vi "Map.vi"(7 "Action":enum8{"noop", "get", "set", "pop"}(ring), 9 "Is Registered in":bool, 10 "User Event in":refnum<user-event>, 11 "User Event Name":string) -> (0 "Found?":bool, 1 "Is Registered out":bool, 2 "User Event out":refnum<user-event>)   [LabVIEW 2018, in "UserEvent.lvlib"]
uses:
  UserEvent.lvlib
panel:
  # "Missing object. The object \"Map\" does not exist in the previous version."
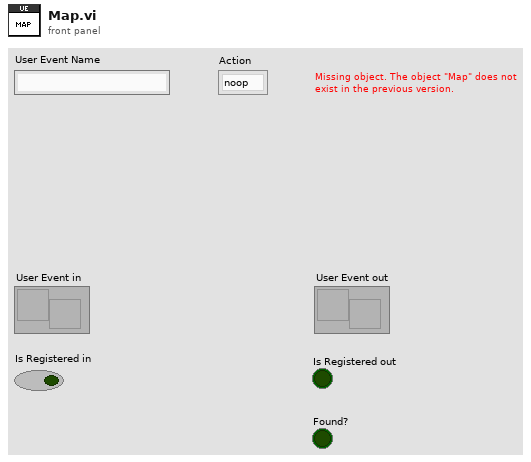
[diagram p1: front panel]
types:
  T1 = cluster{"User Event in":refnum<user-event>, "Is Registered in":bool}
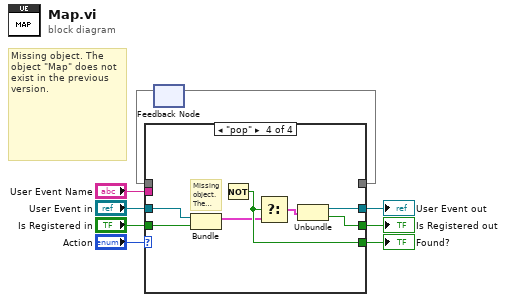
[diagram p0: block diagram]
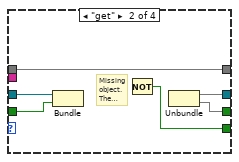
[diagram p3: hidden frame]
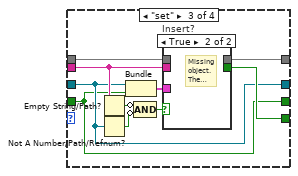
[diagram p4: hidden frame]
diagram:
  # "Missing object. The object \"Map\" does not exist in the previous version."
  n1 = feedback #1() -> (w8, w4)
  n2 = case shown="\"pop\"" "Action" {
    tunnel: [w12 w15 w23 w33] -> w10
    tunnel: "User Event Name" -> [_ w18 w30 w40]
    tunnel: w8 -> [w13 w20 w29 w42]
    tunnel: [w13 w20 w28 w41] -> w7
    tunnel: [_ w17 w24 w36] -> w6
    tunnel: "User Event in" -> [w12 w19 w23 w39]
    tunnel: "Is Registered in" -> [w11 w16 w22 w34]
    tunnel: [w11 w14 w22 w32] -> w1
    frame "noop" {
    }
    frame "get" {
      # "Missing object. The object \"Look In Map\" does not exist in the previous version."
      n3 = Bundle("User Event in"=w19, "Is Registered in"=w16) -> ()  [unwired: 1 in, 1 out]
      n4 = Not() -> (.not. x?=w17:bool)  [unwired: 1 in]
      n5 = Unbundle() -> ("User Event"=w15, "Ready"=w14)  [unwired: 1 in]
    }
    frame "set" {
      n6 = Empty String/Path?(string/path=w30) -> (empty?=w27:bool)
      n7 = Not A Number/Path/Refnum?(number/path/refnum=w23) -> (NaN/Path/Refnum?=w25:bool)
      n8 = Bundle("User Event in"=w23, "Is Registered in"=w22) -> (w21:T1)  [unwired: 1 in]
      n9 = Compound Arithmetic op=AND(invert w27, invert w25) -> (w26:bool)
      n10 = case "Insert?" shown="True" w26 {
        tunnel: w29 -> [w31 _]
        tunnel: w21 -> [_ _]
        tunnel: w30 -> [_ _]
        tunnel: [w31 _] -> w28
        tunnel: [_ _] -> w24
        frame False {
        }
        frame True {
          # "Missing object. The object \"Insert Into Map\" does not exist in the previous version."
        }
      }
    }
    frame "pop" {
      # "Missing object. The object \"Remove From Map\" does not exist in the previous version."
      n11 = Bundle("User Event in"=w39, "Is Registered in"=w34) -> (w35:T1)  [unwired: 1 in]
      n12 = Not() -> (.not. x?=w36:bool)  [unwired: 1 in]
      n13 = Select(s=w36, f=w35) -> (t=w38:T1, s? t:f=w37:T1)
      n14 = Unbundle(w37) -> ("User Event in"=w33:refnum<user-event>, "Is Registered in"=w32:bool)
    }
  }
  "User Event out" <- w10
  "Found?" <- w6
  "Is Registered out" <- w1
  n15 = feedback-in #1(w7) -> ()
